vi "Leds.vi"(1 "R":bool, 2 "G":bool, 3 "B":bool) -> ()   [LabVIEW 2016]
uses:
  <vilib>/Rock Robotics/WPI/Solenoid/WPI_SolenoidValue.ctl
  <vilib>/Rock Robotics/WPI/Solenoid/WPI_SolenoidSetEnum.vi
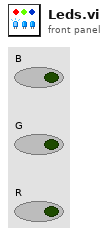
[diagram p1: front panel]
types:
  T1 = typedef "WPI_SolenoidValue.ctl" = enum16{"Off", "On", "Forward", "Reverse"}
  T2 = typedef "WPI_SolenoidDevRef.ctl" = cluster{"DevStatus":errorcluster, "Pneumatics Control Module":u8, "Forward Solenoid Channel":T3, "Reverse Solenoid Channel":T3}
  T3 = typedef "WPI_SolenoidChannel.ctl" = enum8{"Solenoid 0", "Solenoid 1", "Solenoid 2", "Solenoid 3", "Solenoid 4", "Solenoid 5", "Solenoid 6", "Solenoid 7", "Invalid"}
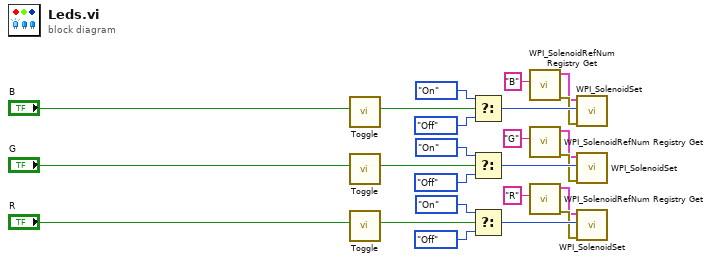
[diagram p0: block diagram]
diagram:
  n1 = call "Toggle.vi"("Input"="B") -> ("Output"=w19:bool)  [unwired: 10 in]
  n2 = call "Toggle.vi"("Input"="G") -> ("Output"=w20:bool)  [unwired: 10 in]
  n3 = call "Toggle.vi"("Input"="R") -> ("Output"=w21:bool)  [unwired: 10 in]
  n4 = Select(t=WPI_SolenoidValue."On" ("Shift Value"), s=w19, f=WPI_SolenoidValue."Off" ("Shift Value")) -> (s? t:f=w10:T1)
  n5 = Select(t=WPI_SolenoidValue."On" ("Shift Value"), s=w20, f=WPI_SolenoidValue."Off" ("Shift Value")) -> (s? t:f=w11:T1)
  n6 = Select(t=WPI_SolenoidValue."On" ("Shift Value"), s=w21, f=WPI_SolenoidValue."Off" ("Shift Value")) -> (s? t:f=w12:T1)
  n7 = call <vilib>:"WPI_SolenoidRefNum Registry Get.vi"("refnum name"="B") -> ("error out"=w5:errorcluster, "SolenoidDevRef"=w4:T2)  [unwired: 9 in]
  n8 = call <vilib>:"WPI_SolenoidRefNum Registry Get.vi"("refnum name"="G") -> ("error out"=w7:errorcluster, "SolenoidDevRef"=w6:T2)  [unwired: 9 in]
  n9 = call <vilib>:"WPI_SolenoidRefNum Registry Get.vi"("refnum name"="R") -> ("error out"=w9:errorcluster, "SolenoidDevRef"=w8:T2)  [unwired: 9 in]
  n10 = call-poly <vilib>:"WPI_SolenoidSet.vi"("error in (no error)"=w5, "Value"=w10, "SolenoidDevRef"=w4) -> ()  [unwired: 7 in, 2 out]
  n11 = call-poly <vilib>:"WPI_SolenoidSet.vi"("error in (no error)"=w7, "Value"=w11, "SolenoidDevRef"=w6) -> ()  [unwired: 7 in, 2 out]
  n12 = call-poly <vilib>:"WPI_SolenoidSet.vi"("error in (no error)"=w9, "Value"=w12, "SolenoidDevRef"=w8) -> ()  [unwired: 7 in, 2 out]
